vi "ExpandPic.vi"(2 "Colored bitmap":i32[][](array[numeric]), 3 "Picture in":refnum<vi>) -> (0 "Expand test pic. 2":picture caption="Expand pic.", 1 "Debug test pic.":picture caption="Debug  pic.")   [LabVIEW 2016]
panel:
  out "new picture":picture
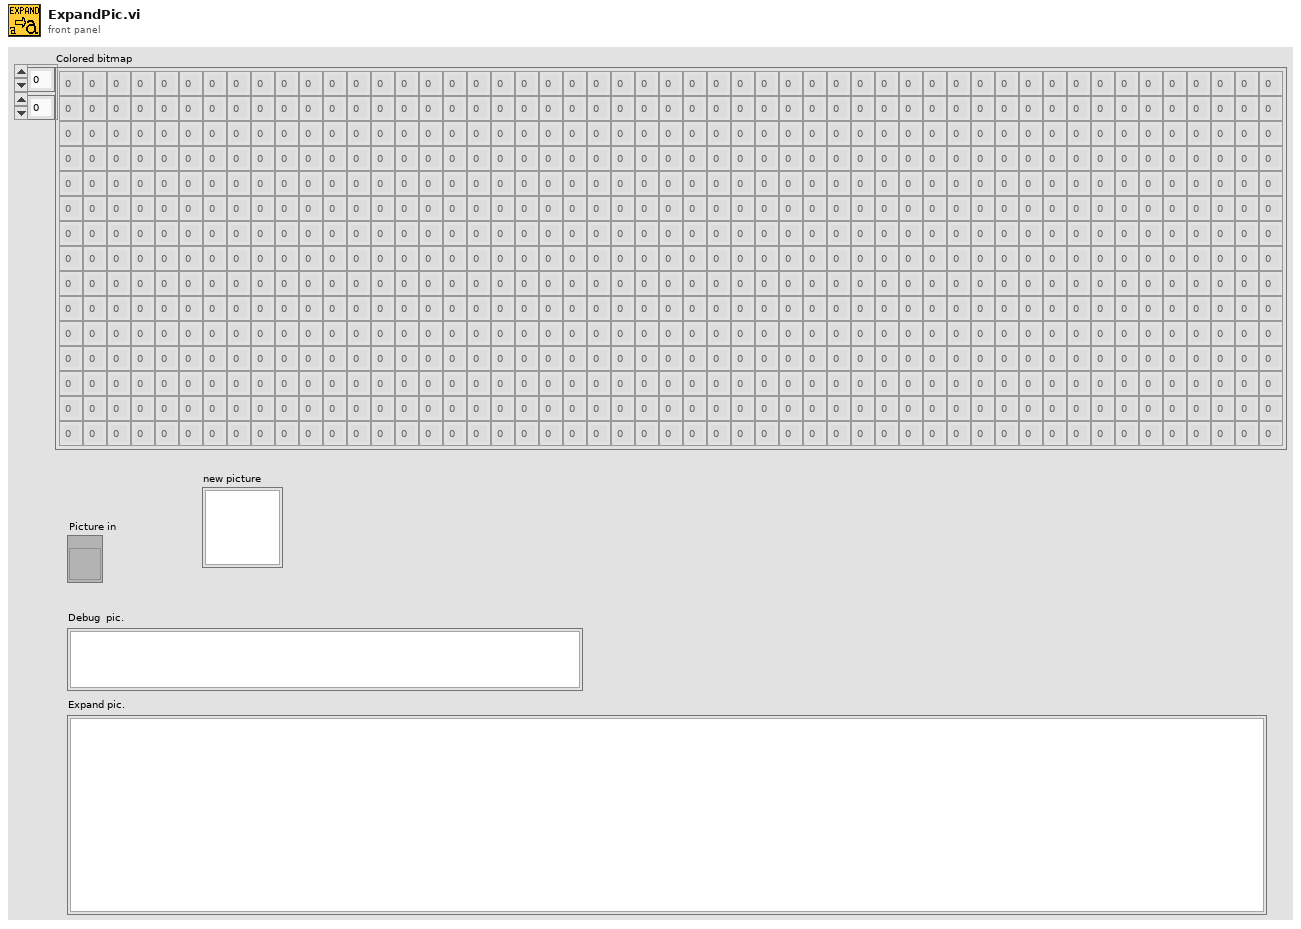
[diagram p1: front panel]
types:
  T1 = typedef "imagedata.ctl" = cluster{"image type":i32, "image depth":i32, "image":u8[], "mask":u8[], "colors":u32[], "Rectangle":cluster{"left":i16, "top":i16, "right":i16, "bottom":i16}}
  T2 = typedef "LVBoundsTypeDef.ctl" = cluster{"Width":u32, "Height":u32}
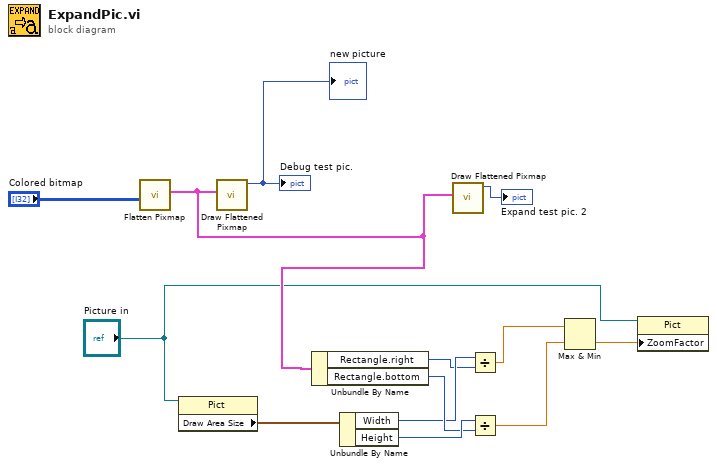
[diagram p0: block diagram]
diagram:
  n1 = call <vilib>:"Flatten Pixmap.vi"("4-bit pixmap"="Colored bitmap") -> ("image data"=w11:T1)  [unwired: 10 in]
  n2 = property on="Property Node" class="Pict"(reference="Picture in") -> ("Draw Area Size"=w2:T2)  [unwired: 1 in, 2 out]
  n3 = call <vilib>:"Draw Flattened Pixmap.vi"("image data"=w11) -> ("new picture"=→"Debug test pic." →"new picture":picture)  [unwired: 8 in]
  n4 = Unbundle By Name(w11) -> ("Rectangle.right"=w3:i16, "Rectangle.bottom"=w5:i16)
  n5 = Unbundle By Name(w2) -> ("Width"=w4:u32, "Height"=w6:u32)
  n6 = call <vilib>:"Draw Flattened Pixmap.vi"("image data"=w11) -> ("new picture"=→"Expand test pic. 2":picture)  [unwired: 8 in]
  n7 = Divide(x=w4, y=w3) -> (x/y=w8:dbl)
  n8 = Divide(x=w6, y=w5) -> (x/y=w7:dbl)
  n9 = Max & Min(x=w8, y=w7) -> (min(x,y)=w9:dbl)  [unwired: 1 out]
  n10 = property on="Property Node" class="Pict"(reference="Picture in", "ZoomFactor"=w9) -> ()  [unwired: 1 in, 2 out]
